vi "Del graph.vi"(8 "error in (no error)":errorcluster, 9 "selected graph":i32, 10 "Combo Box":string(combo)="Kinetics", 11 "Control-Client in":refnum<class "Control-Client.lvclass">) -> (0 "error out":errorcluster, 3 "Control-Client out":refnum<class "Control-Client.lvclass">)   [LabVIEW 2018, in "Control-Client.lvclass"]
uses:
  Control-Client.lvclass
  Control-Client.lvclass/Control-Client.ctl
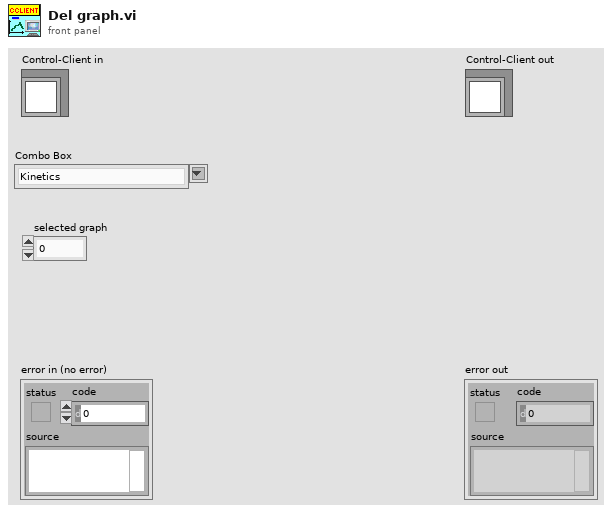
[diagram p1: front panel]
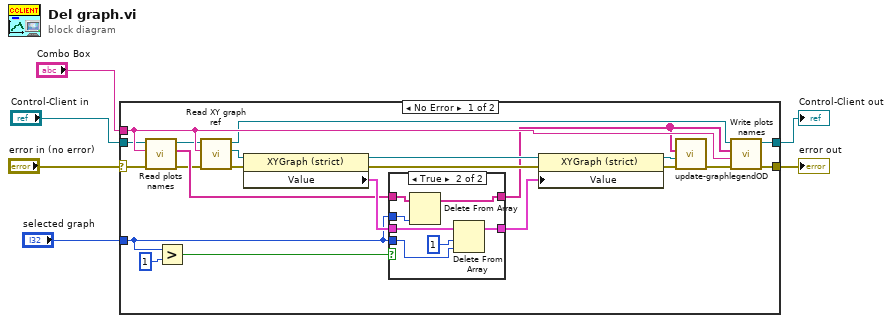
[diagram p0: block diagram]
diagram:
  n1 = case shown="No Error" "error in (no error)" {
    selector: "error in (no error)" -> [w14 w39]
    tunnel: [w7 w39] -> w5
    tunnel: [w18 w38] -> w3
    tunnel: "Control-Client in" -> [w10 w38]
    tunnel: "selected graph" -> [w21 _]
    tunnel: "Combo Box" -> [w20 _]
    frame No Error {
      n2 = call "Read plots names.vi"("error in (no error)"=w14, "Combo Box"=w20, "Control-Client in"=w10) -> ("error out"=w13:errorcluster, "Plots names"=w22:string[], "Control-Client out"=w12:refnum<class "Control-Client.lvclass">)  [unwired: 6 in]
      n3 = Greater?(x=w21, y=1) -> (0:w28:bool)
      n4 = call "Read XY graph ref.vi"("error in (no error)"=w13, "Combo Box"=w20, "Control-Client in"=w12) -> ("error out"=w19:errorcluster, "XY graph ref"=w17:refnum<vi>, "Control-Client out"=w11:refnum<class "Control-Client.lvclass">)  [unwired: 6 in]
      n5 = property class="XYGraph (strict)"(reference=w17, error in=w19) -> (reference out=w24:refnum<vi>, error out=w23:errorcluster, "Value"=w26:cluster{"Y":dbl[], "Y":dbl[]}[])
      n6 = case shown="True" w28 {
        tunnel: [w30 w37] -> w25
        tunnel: w21 -> [_ w34]
        tunnel: w21 -> [_ w35]
        tunnel: w26 -> [w30 w33]
        tunnel: w22 -> [w29 w32]
        tunnel: [w29 w31] -> w15
        frame False {
        }
        frame True {
          n7 = Delete From Array(array=w32, index=w35) -> (array with subset deleted=w31:string[])  [unwired: 1 in, 1 out]
          n8 = Delete From Array(array=w33, length=1, index=w34) -> (array with subset deleted=w37:cluster{"Y":dbl[], "Y":dbl[]}[])  [unwired: 1 out]
        }
      }
      n9 = property class="XYGraph (strict)"(reference=w24, error in=w23, "Value"=w25) -> (reference out=w16:refnum<vi>, error out=w9:errorcluster)
      n10 = call "update-graphlegendOD.vi"("error in (no error)"=w9, "XYGraph in"=w16, "plot names"=w15) -> ("error out"=w8:errorcluster)  [unwired: 7 in]
      n11 = call "Write plots names.vi"("error in (no error)"=w8, "Combo Box"=w20, "Plot names"=w15, "Control-Client in"=w11) -> ("error out"=w7:errorcluster, "Control-Client out"=w18:refnum<class "Control-Client.lvclass">)  [unwired: 6 in]
    }
    frame Error {
    }
  }
  "error out" <- w5
  "Control-Client out" <- w3
